vi "Clone.vi"(6 "Error on existing directory":bool=TRUE caption="Error on existing directory? (T)", 8 "error in (no error)":errorcluster, 9 "Remote URL":string, 10 "Target Directory":path, 11 "Git Implementation in":refnum<class "Git Implementation.lvclass">) -> (0 "error out":errorcluster, 2 "Status Message":string, 3 "Git Implementation out":refnum<class "Git Implementation.lvclass">)   [LabVIEW 2017, in "Git Implementation.lvclass"]
doc: "Clone a repository from the Remote URL.\nThe repository will be cloned into the directory specified as the Target Directory, which should be either nonexistent or empty.\nDo not use the Status Message as a parseable output - it is for user information/display only and may change between versions."
uses:
  Git Implementation.lvclass
  Git Implementation.lvclass/Git Implementation.ctl
  <vilib>/Utility/error.llb/Error Cluster From Error Code.vi
  <vilib>/ErrorRing/Error Ring.xnode
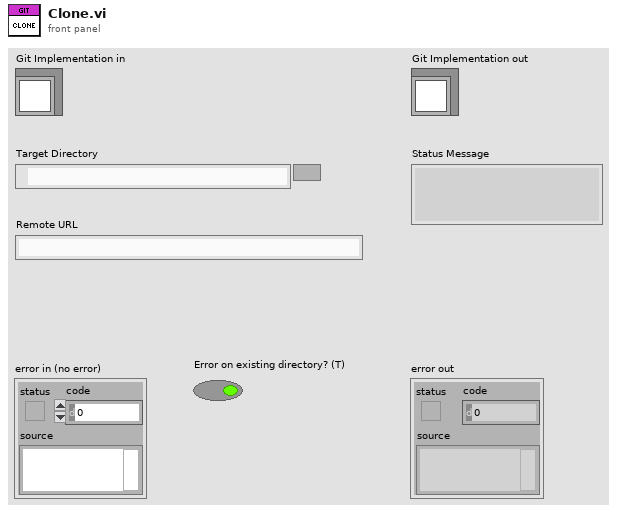
[diagram p1: front panel]
types:
  T1 = typedef "Git Implementation.lvclass/CMD Return.ctl" = cluster{"StdOut":string, "StdErr":string, "Return Code":i32}
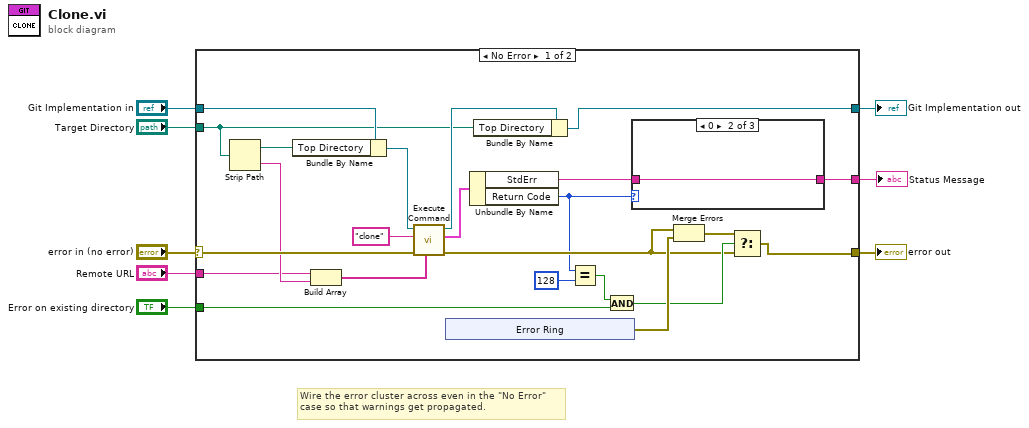
[diagram p0: block diagram]
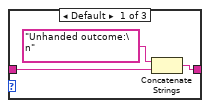
[diagram p2: hidden frame]
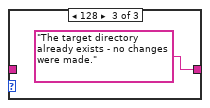
[diagram p3: hidden frame]
diagram:
  # "Wire the error cluster across even in the \"No Error\"\ncase so that warnings get propagated."
  n1 = case shown="No Error" "error in (no error)" {
    selector: "error in (no error)" -> [w30 w42]
    tunnel: [w14 w42] -> w7
    tunnel: [w22 w41] -> w5
    tunnel: "Git Implementation in" -> [w29 w41]
    tunnel: "Target Directory" -> [w21 _]
    tunnel: "Remote URL" -> [w23 _]
    tunnel: "Error on existing directory" -> [w16 _]
    tunnel: [w10 _] -> w1
    frame No Error {
      n2 = Strip Path(path=w21) -> (stripped path=w28:path, name=w24:string)
      n3 = Bundle By Name(cluster=w29, "Top Directory"=w28) -> (w27:refnum<class "Git Implementation.lvclass">)
      n4 = Build Array(w23, w24) -> (w20:string[])
      n5 = call "Execute Command.vi"("Arguments"=w20, "error in (no error)"=w30, "Command"="clone", "Git Implementation in"=w27) -> ("error out"=w13:errorcluster, "CMD Return"=w19:T1, "Git Implementation out"=w26:refnum<class "Git Implementation.lvclass">)  [unwired: 5 in]
      n6 = xnode "Error Ring"() -> ("error out"=w31:errorcluster)
      n7 = Unbundle By Name(w19) -> ("StdErr"=w9:string, "Return Code"=w11:i32)
      n8 = Bundle By Name(cluster=w26, "Top Directory"=w21) -> (w22:refnum<class "Git Implementation.lvclass">)
      n9 = Equal?(x=w11, y=128) -> (x = y?=w17:bool)
      n10 = And(x=w17, y=w16) -> (x .and. y?=w15:bool)
      n11 = case shown="0" w11 {
        tunnel: [w38 w39 "The target directory already exists - no changes were made."] -> w10
        tunnel: w9 -> [w37 w39 _]
        frame Default {
          n12 = Concatenate Strings("Unhanded outcome:\n" ("string"), w37) -> (w38:string)
        }
        frame 0 {
        }
        frame 128 {
        }
      }
      n13 = Merge Errors(w13, w31) -> (w12:errorcluster)
      n14 = Select(t=w12, s=w15, f=w13) -> (s? t:f=w14:errorcluster)
    }
    frame Error {
    }
  }
  "error out" <- w7
  "Git Implementation out" <- w5
  "Status Message" <- w1
